vi "lab5.vi"() -> ()   [LabVIEW 2020]
panel:
  out "Waveform Chart 3":dbl(graph)
  out "Waveform Chart 2":dbl(graph)
  out "Waveform Chart":dbl(graph)
  out "Array":dbl[](array[numeric])
  in  "C":dbl
  out "Время разрядки":dbl
  out "Сила тока":dbl
  out "Заряд":dbl
  in  "Остаточное напряжение":dbl
  in  "R":dbl
  in  "ЭДС":dbl
  out "C voltage":dbl(knob) scale=0.0..10.0
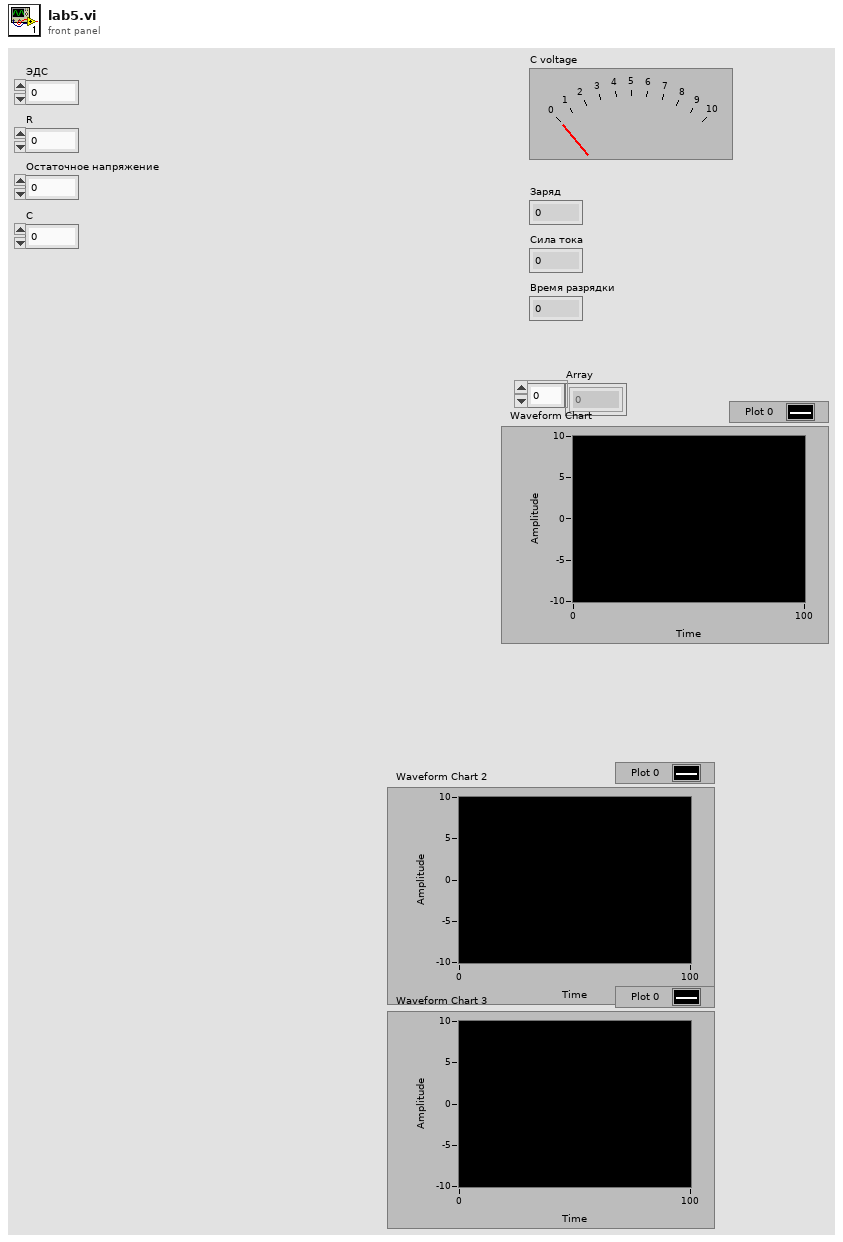
[diagram p1: front panel]
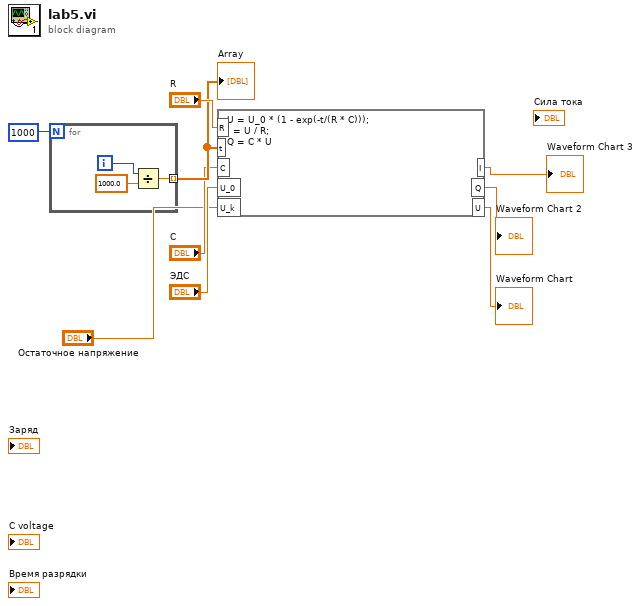
[diagram p0: block diagram]
diagram:
  n1 = for {
    N: 1000 -> [_]
    tunnel: [w10] -> w7 mode=indexing
    i -> [w11]
    n2 = Divide(x=w11, y=1000.0) -> (x/y=w10:dbl)
  }
  "Array" <- w7
  n3 = formula code="U = U_0 * (1 - exp(-t/(R * C)));\nI = U / R;\nQ = C * U"("R"="R", "t"=w7, "C"="C", "U_0"="ЭДС", "U_k"="Остаточное напряжение") -> ("I"=→"Waveform Chart 3":dbl, "Q"=→"Waveform Chart 2":dbl, "U"=→"Waveform Chart":dbl)
